vi "EnablePositionWindow.vi"(4 "error in (no error)":errorcluster, 6 "position window":T1, 7 "axis in":cluster{"keyHandle":u32, "nodeId":u16}={"keyHandle"=0, "nodeId"=1}) -> (0 "error out":errorcluster, 3 "axis out":cluster{"keyHandle":u32, "nodeId":u16}={"keyHandle"=0, "nodeId"=1})   [LabVIEW 2010]
doc: "<B>VCS_EnablePositionWindow</B> activates the position window."
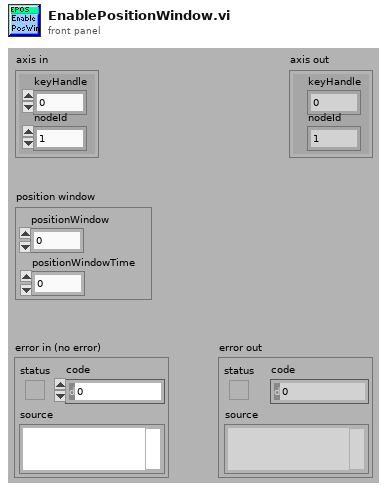
[diagram p1: front panel]
types:
  T1 = cluster{"positionWindow":u32, "positionWindowTime":u16}
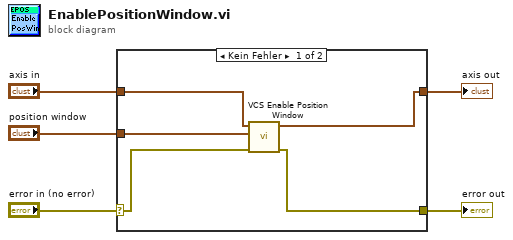
[diagram p0: block diagram]
diagram:
  n1 = case shown="Kein Fehler" "error in (no error)" {
    selector: "error in (no error)" -> [w10 w12]
    tunnel: [w9 w12] -> w4
    tunnel: [w8 w11] -> w3
    tunnel: "axis in" -> [w7 w11]
    tunnel: "position window" -> [w6 _]
    frame No Error {
      n2 = call "VCS Enable Position Window.vi"("error in (no error)"=w10, "position window"=w6, "axis in"=w7) -> ("error out"=w9:errorcluster, "axis out"=w8:cluster{"keyHandle":u32, "nodeId":u16})  [unwired: 7 in]
    }
    frame Error {
    }
  }
  "error out" <- w4
  "axis out" <- w3
